vi "Set Fixed-Point Information.vi"(6 "Include Overflow Status?":bool, 8 "error in (no error)":errorcluster, 9 "FXP Range":T1, 10 "FXP Representation":T2, 11 "Variant in":variant) -> (0 "error out":errorcluster, 3 "Variant out":variant)   [LabVIEW 2020, in "NI_Data Type.lvlib"]
doc: "Sets the attributes of a fixed-point numeric data type.\n\nVariant in - the fixed-point numeric data type whose attributes will be set. If any attributes already exist, they will be overwritten.\nFXP Representation - the new FXP representation.\nFXP Range - the new FXP range.\nInclude Overflow Status - the new overflow status.\nVariant out - the resulting fixed-point numeric type."
uses:
  <vilib>/Utility/Data Type/NI_Data Type.lvlib
  <vilib>/fxp/LVFixedPointRepBitsTypeDef.ctl
  <vilib>/fxp/LVFixedPointRepRangeTypeDef.ctl
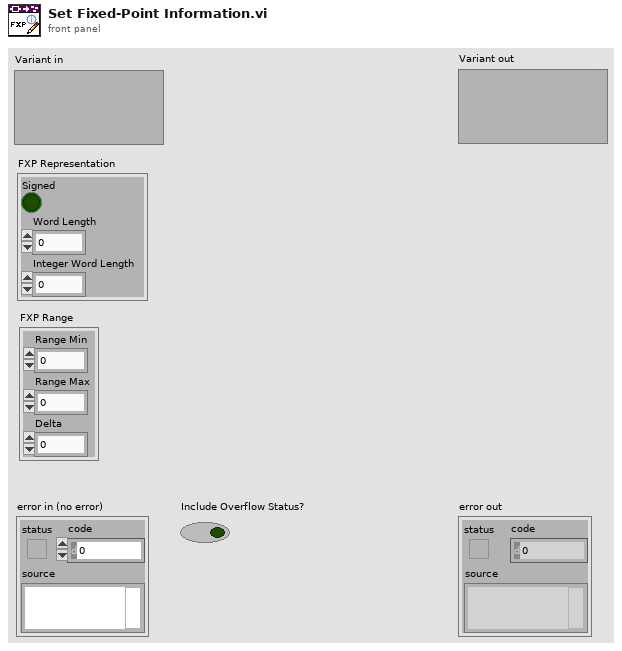
[diagram p1: front panel]
types:
  T1 = typedef "LVFixedPointRepRangeTypeDef.ctl" = cluster{"Range Min":dbl, "Range Max":dbl, "Delta":dbl}
  T2 = typedef "LVFixedPointRepBitsTypeDef.ctl" = cluster{"Signed":bool, "Word Length":u32, "Integer Word Length":i32}
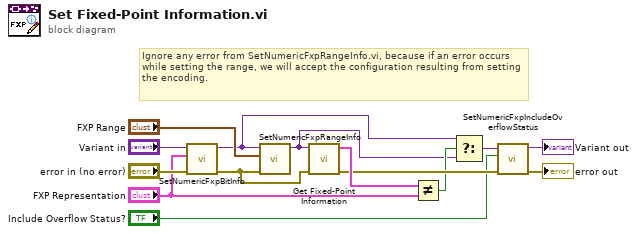
[diagram p0: block diagram]
diagram:
  # "Ignore any error from SetNumericFxpRangeInfo.vi, because if an error occurs while setting the range, we will accept the configuration resulting from setting the encoding."
  n1 = call <vilib>:"SetNumericFxpBitInfo.vi"("error in (no error)"="error in (no error)", "FXP Representation"="FXP Representation", "Variant in"="Variant in") -> ("error out"=w9:errorcluster, "Variant out"=w2:variant)  [unwired: 7 in]
  n2 = call <vilib>:"SetNumericFxpRangeInfo.vi"("error in (no error)"=w9, "FXP Range"="FXP Range", "Variant in"=w2) -> ("Variant out"=w1:variant)  [unwired: 7 in, 1 out]
  n3 = call <vilib>:"Get Fixed-Point Information.vi"("error in (no error)"=w9, "variant"=w1) -> ("error out"=w7:errorcluster, "FXP representation"=w10:T2)  [unwired: 6 in, 2 out]
  n4 = Not Equal?(x=w10, y="FXP Representation") -> (x != y?=w4:bool)
  n5 = Select(t=w2, s=w4, f=w1) -> (s? t:f=w3:variant)
  n6 = call <vilib>:"SetNumericFxpIncludeOverflowStatus.vi"("error in (no error)"=w7, "Include Overflow Status?"="Include Overflow Status?", "Variant in"=w3) -> ("error out"=→"error out":errorcluster, "Variant out"=→"Variant out":variant)  [unwired: 7 in]
